vi "Read Listener.vi"(8 "Error In":errorcluster, 11 "Listener ID":string) -> (0 "Error Out":errorcluster, 3 "Listener":refnum<queue>)   [LabVIEW 2018, in "Toolkit.lvlib"]
doc: "Gets the logging statements for a listener."
uses:
  Toolkit.lvlib
  Type Definitions/Statement.ctl
  Type Definitions/Tag.ctl
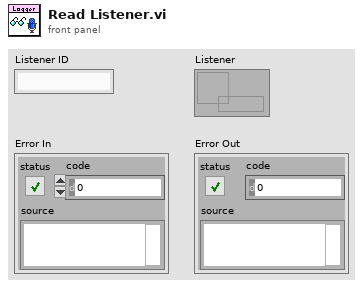
[diagram p1: front panel]
types:
  T1 = typedef "Toolkit.lvlib/Statement.ctl" = cluster{"Time Stamp":timestamp, "Tag":T2, "Source":string, "Message":string}
  T2 = typedef "Toolkit.lvlib/Tag.ctl" = enum16{"Fatal", "Error", "Warn", "Info", "Debug", "Trace"}
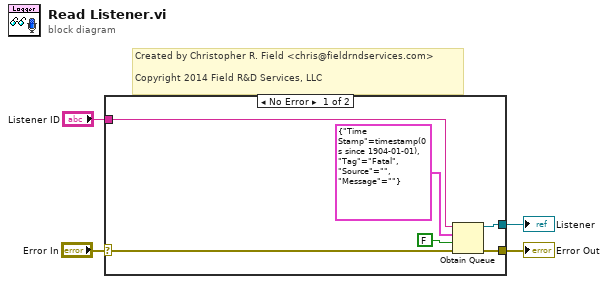
[diagram p0: block diagram]
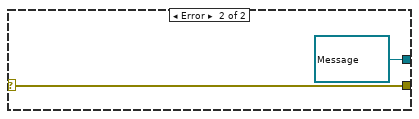
[diagram p2: hidden frame]
diagram:
  # "Created by Christopher R. Field <chris@fieldrndservices.com>\n\nCopyright 2014 Field R&D Services, LLC"
  n1 = case shown="No Error" "Error In" {
    selector: "Error In" -> [w8 w12]
    tunnel: "Listener ID" -> [w9 _]
    tunnel: [w7 w12] -> w2
    tunnel: [w6 refnum<queue> refnum ("queue out")] -> w1
    frame No Error {
      n2 = Obtain Queue(name (unnamed)=w9, element data type=T1 {"Time Stamp"=timestamp(0 s since 1904-01-01), "Tag"=enum."Fatal", "Source"="", "Message"=""} ("Message"), create if not found? (T)=FALSE, error in (no error)=w8) -> (queue out=w6:refnum<queue>, error out=w7:errorcluster)  [unwired: 1 in, 1 out]
    }
    frame Error {
    }
  }
  "Error Out" <- w2
  "Listener" <- w1
